vi "Annotations Tip Strip Data FGV.vi"(1 "Action(GET)":T3(ring), 7 "Annotations Tip Strip Data in":T1, 11 "error in (no error)":errorcluster) -> (8 "Annotations Tip Strip Data in":T1, 15 "error out":errorcluster)   [LabVIEW 2011]
uses:
  Annotations Tip Strip FGV_data cluster.ctl
  <vilib>/Utility/miscctls.llb/LVPoint32TypeDef.ctl
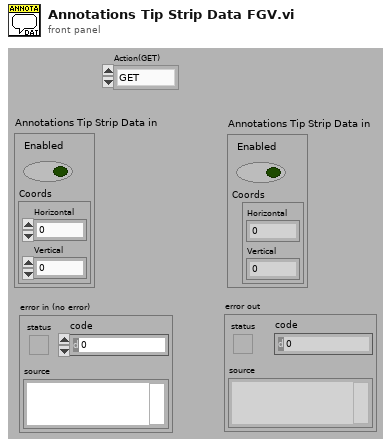
[diagram p1: front panel]
types:
  T1 = typedef "Annotations Tip Strip FGV_data cluster.ctl" = cluster{"Enabled":bool, "Point32":T2}
  T2 = typedef "LVPoint32TypeDef.ctl" = cluster{"Horizontal":i32, "Vertical":i32}
  T3 = enum16{"GET", "SET", "Get from Ini", "Put in Ini"}
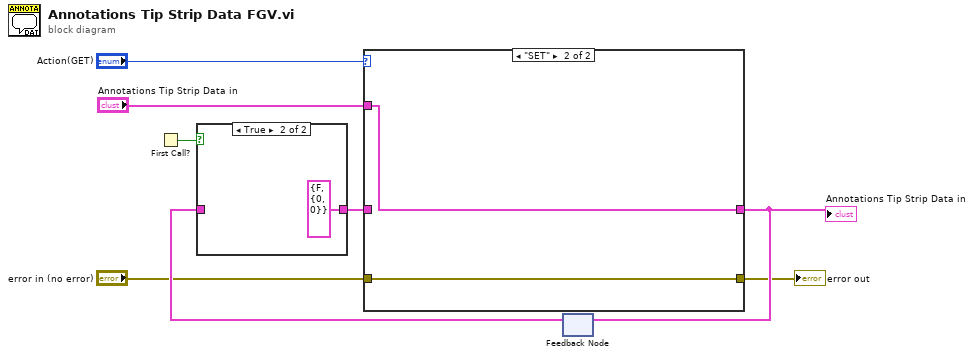
[diagram p0: block diagram]
diagram:
  n1 = First Call?() -> (First Call?: T/F=w7:bool)
  n2 = feedback #1() -> (w8:T1)  [unwired: 1 in]
  n3 = case shown="True" w7 {
    tunnel: w8 -> [w9 _]
    tunnel: [w9 T1 {"Enabled"=FALSE, "Point32"={"Horizontal"=0, "Vertical"=0}} ("Annotations Tip Strip Data in")] -> w5
    frame False {
    }
    frame True {
    }
  }
  n4 = case shown="\"SET\"" "Action(GET)" {
    tunnel: [w12 w14] -> w6
    tunnel: w5 -> [w12 _]
    tunnel: "Annotations Tip Strip Data in" -> [_ w14]
    tunnel: "error in (no error)" -> [w11 w13]
    tunnel: [w11 w13] -> w1
    frame "GET", Default {
    }
    frame "SET" {
    }
  }
  "error out" <- w1
  "Annotations Tip Strip Data in" <- w6
  n5 = feedback-in #1(w6) -> ()
